vi "digital_io_test.vi"() -> ()   [LabVIEW 2010]
uses:
  <vilib>/Utility/error.llb/DialogType.ctl
  <vilib>/DAQmx/read.llb/DAQmx Read (Analog Wfm 1Chan NSamp).vi
  <vilib>/DAQmx/write.llb/DAQmx Write (Digital 1D Bool 1Chan 1Samp).vi
  <vilib>/DAQmx/create/channels.llb/DAQmx Create Channel (DO-Digital Output).vi
  <vilib>/DAQmx/create/channels.llb/DAQmx Create Channel (AI-Voltage-Basic).vi
  <vilib>/DAQmx/configure/timing.llb/DAQmx Timing (Sample Clock).vi
  <vilib>/DAQmx/configure/trigger.llb/DAQmx Start Trigger (Digital Edge).vi
  <vilib>/daqmx/miscellaneous.llb/DAQmx Fill In Error Info.vi
panel:
  out "data":waveform(dbl)
  in  "physical channels":tag
  in  "stop":bool
  in  "Data to Write":bool[](array[boolean])=[FALSE, FALSE, FALSE, FALSE, FALSE, FALSE, FALSE, FALSE]
  in  "Lines":tag="Dev1/port0/line0:7"
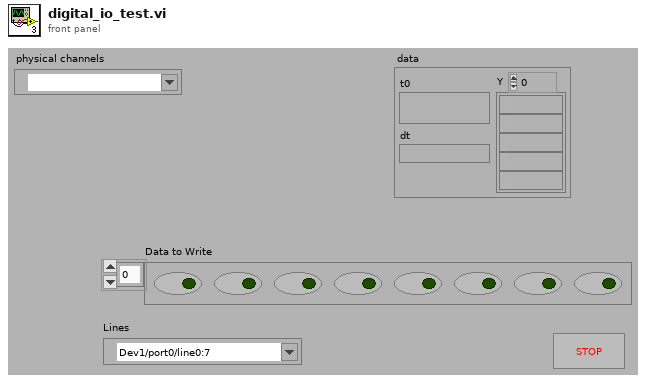
[diagram p1: front panel]
types:
  T1 = typedef "DialogType.ctl" = u16
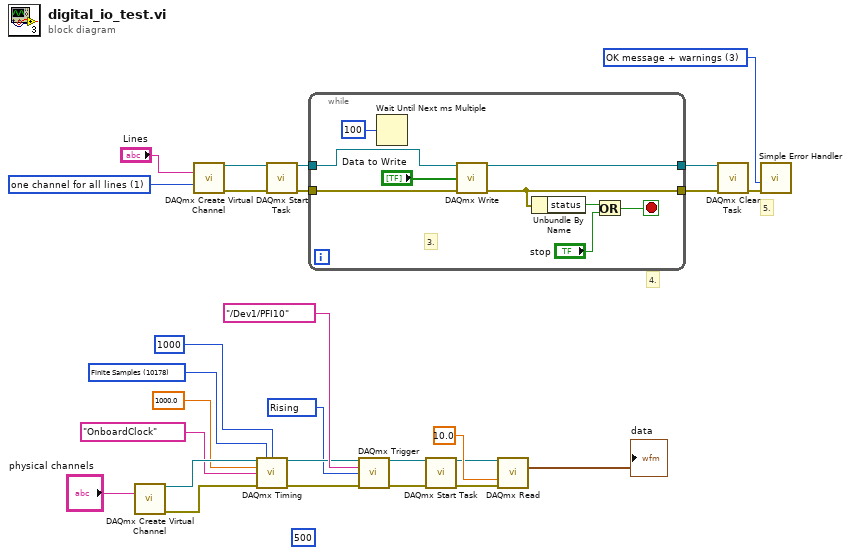
[diagram p0: block diagram]
diagram:
  w5 = 10178 items=["Finite Samples"=10178, "Continuous Samples"=10123, "Hardware Timed Single Point"=12522] ("sample mode")
  w8 = 10280 items=["Rising"=10280, "Falling"=10171] ("edge")
  (unwired) u32 500 ("pretrigger samples per channel")
  w21 = T1 3 items=["no dialog", "OK message", "continue or stop message", "OK message + warnings", "continue/stop + warnings"] ("type of dialog (OK msg:1)")
  w25 = 1 items=["one channel for each line", "one channel for all lines"] ("line grouping")
  # "5."
  # "4."
  n1 = call-poly <vilib>:"DAQmx Create Virtual Channel.vi"("physical channels"="physical channels") -> ("task out"=w13:refnum<k21>, "error out"=w10:errorcluster)  [unwired: 13 in]
  n2 = call-poly <vilib>:"DAQmx Create Virtual Channel.vi"("lines"="Lines", "line grouping"=w25) -> ("task out"=w27:refnum<k21>, "error out"=w26:errorcluster)  [unwired: 12 in]
  n3 = call-poly <vilib>:"DAQmx Timing.vi"("task/channels in"=w13, "sample mode"=w5, "samples per channel"=1000, "rate"=1000.0, "source"=tag "OnboardClock", "error in"=w10) -> ("task out"=w12:refnum<k21>, "error out"=w11:errorcluster)  [unwired: 8 in]
  n4 = call <vilib>:"DAQmx Start Task.vi"("task/channels in"=w27, "error in"=w26) -> ("task out"=w20:refnum<k21>, "error out"=w19:errorcluster)  [unwired: 12 in]
  n5 = while {
    tunnel: w19 -> [w36]
    tunnel: [w32] -> w24
    tunnel: w20 -> [w31]
    tunnel: [w30] -> w22
    stop <- w35 stop-if-true
    # "3."
    n6 = Wait Until Next ms Multiple(millisecond multiple=u32 100 ("milliseconds to wait")) -> ()  [unwired: 1 out]
    n7 = call-poly <vilib>:"DAQmx Write.vi"("task/channels in"=w31, "data"="Data to Write", "error in"=w36) -> ("task out"=w30:refnum<k21>, "error out"=w32:errorcluster)  [unwired: 10 in, 1 out]
    n8 = Unbundle By Name(w32) -> ("status"=w33:bool)
    n9 = Or(x=w33, y="stop") -> (x .or. y?=w35:bool)
  }
  n10 = call-poly <vilib>:"DAQmx Trigger.vi"("task/channels in"=w12, "source"=tag "/Dev1/PFI10", "edge"=w8, "error in"=w11) -> ("task out"=w16:refnum<k21>, "error out"=w15:errorcluster)  [unwired: 10 in]
  n11 = call <vilib>:"DAQmx Start Task.vi"("task/channels in"=w16, "error in"=w15) -> ("task out"=w3:refnum<k21>, "error out"=w2:errorcluster)  [unwired: 12 in]
  n12 = call-poly <vilib>:"DAQmx Read.vi"("task/channels in"=w3, "timeout"=10.0, "error in"=w2) -> ("data"=→"data":waveform(dbl))  [unwired: 10 in, 2 out]
  n13 = call <vilib>:"DAQmx Clear Task.vi"("task in"=w22, "error in"=w24) -> ("error out"=w23:errorcluster)  [unwired: 13 in]
  n14 = call <vilib>:"Simple Error Handler.vi"("type of dialog (OK msg:1)"=w21, "error in (no error)"=w23) -> ()  [unwired: 3 in, 5 out]
